vi "W7X-Bolo-Timer.vi"(10 "Wait-Time until Trigger\npublished on CODA\ntypically 10 s":u32, 11 "Digital in":refnum<vi>) -> ()   [LabVIEW 2014]
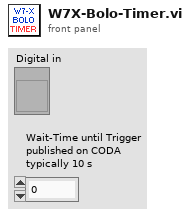
[diagram p1: front panel]
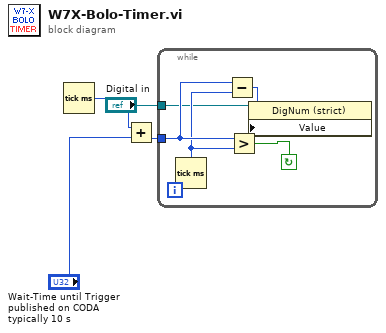
[diagram p0: block diagram]
diagram:
  n1 = Tick Count (ms)() -> (millisecond timer value=w2:u32)
  n2 = Add(x=w2, y="Wait-Time until Trigger\npublished on CODA\ntypically 10 s") -> (x+y=w3:u32)
  n3 = while {
    tunnel: w3 -> [w8]
    tunnel: "Digital in" -> [w5]
    stop <- w9 continue-if-true
    n4 = Tick Count (ms)() -> (millisecond timer value=w7:u32)
    n5 = Subtract(x=w8, y=w7) -> (x-y=w6:u32)
    n6 = Greater?(x=w8, y=w7) -> (0:w9:bool)
    n7 = property class="DigNum (strict)"(reference=w5, "Value"=w6) -> ()  [unwired: 1 in, 2 out]
  }
